vi "Data Cluster.vi"(0 "DAQ Data":dbl, 1 "seconds since 1Jan1904":timestamp, 2 "Array":i32[](array[numeric]), 10 "Cluster in":T1) -> (14 "Cluster out":T1)   [LabVIEW 2017]
uses:
  DAQData.ctl
panel:
  in  "Frequency":dbl
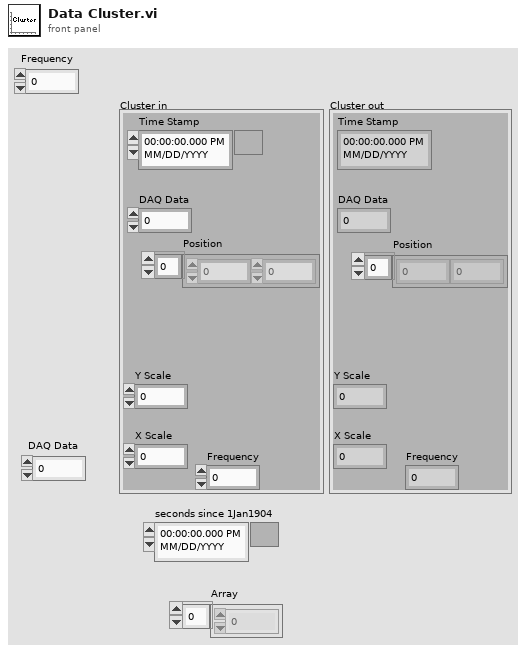
[diagram p1: front panel]
types:
  T1 = typedef "DAQData.ctl" = cluster{"DAQ Data":dbl, "Time Stamp":timestamp, "Y Scale":dbl, "X Scale":dbl, "Position":i32[], "Frequency":dbl}
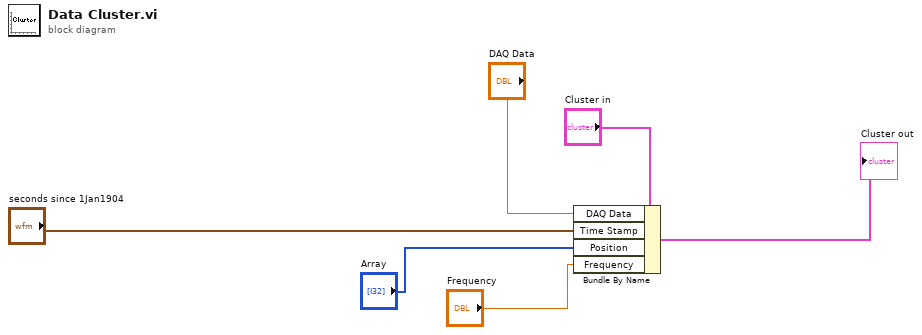
[diagram p0: block diagram]
diagram:
  n1 = Bundle By Name(cluster="Cluster in", "DAQ Data"="DAQ Data", "Time Stamp"="seconds since 1Jan1904", "Position"="Array", "Frequency"="Frequency") -> (→"Cluster out":T1)
